vi "INI-FGV(lvlibp).vi"(4 "Raw String? (F)":bool, 5 "Write If not found?":bool, 6 "Enum":T3, 7 "Prefered Section":string, 8 "error IN":errorcluster, 9 "Path":path, 10 ">> Default Value >>":string, 11 ">> Variable Name >>":string) -> (0 "error out":errorcluster, 1 "INIConfig":T1, 2 "Key?":bool, 3 "Array":string[](array[string]))   [LabVIEW 2017, in "INI-Static-Variable-Support.lvlib"]
uses:
  INI-Static-Variable-Support.lvlib
  _fgv-oper.ctl
  LabVIEW-Config/Config.ctl
  LabVIEW-Config/LineToken.ctl
  INI-FGV.vi
  <userlib>/_NEVSTOP/Communicable State Machine(CSM)/Communicable State Machine.lvlib
  <userlib>/_NEVSTOP/Communicable State Machine(CSM)/_Shared/CSM Shared.lvlib
  LabVIEW-Config/LabVIEW-Config.lvlib
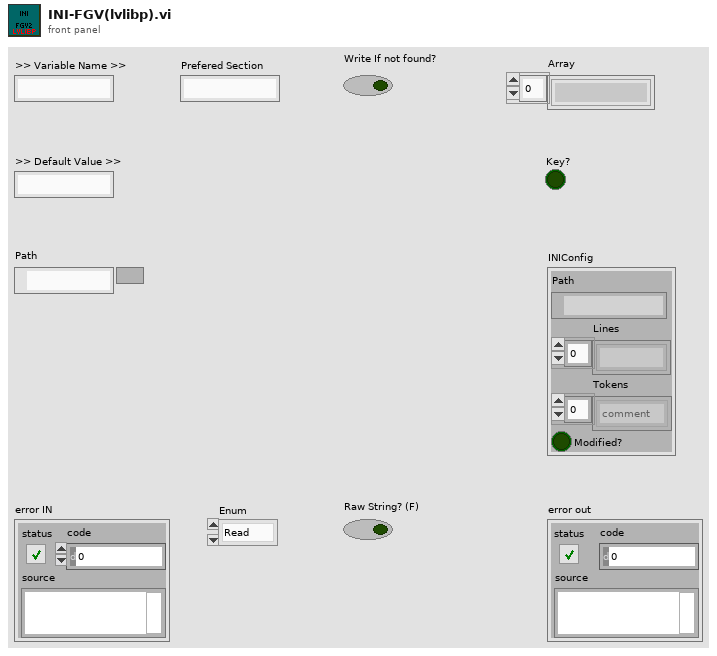
[diagram p1: front panel]
types:
  T1 = typedef "LabVIEW-Config.lvlib/Config.ctl" = cluster{"Path":path, "Lines":string[], "Tokens":T2[], "Modified?":bool}
  T2 = typedef "LabVIEW-Config.lvlib/LineToken.ctl" = enum8{"comment", "section", "key", "more"}
  T3 = typedef "INI-Static-Variable-Support.lvlib/_fgv-oper.ctl" = enum16{"Read", "Write", "Sync", "Sessions", "List Keys", "Load", "List Files", "List Variables", "List Permanent Variables", "Mark Temp Variable as Permenent", "unload", "INIConfig(Memory)", "Reset", "Restore Variable Value"}
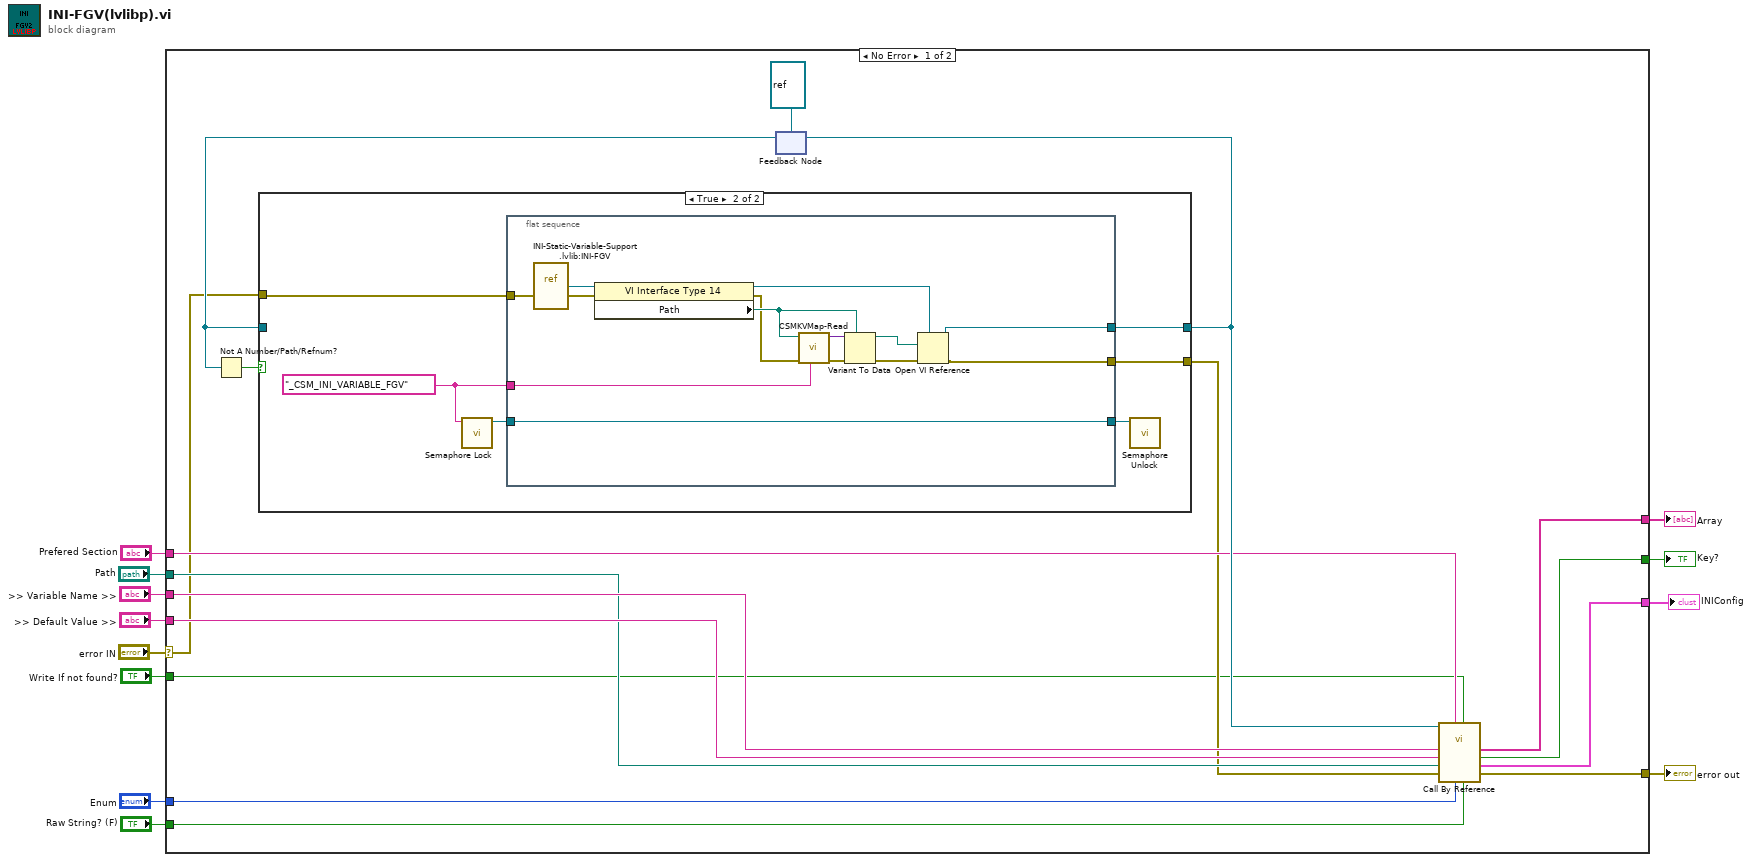
[diagram p0: block diagram]
diagram:
  n1 = case shown="No Error" "error IN" {
    selector: "error IN" -> [w20 w51]
    tunnel: ">> Default Value >>" -> [w23 _]
    tunnel: ">> Variable Name >>" -> [w24 _]
    tunnel: [w16 w51] -> w10
    tunnel: "Enum" -> [w22 _]
    tunnel: "Raw String? (F)" -> [w13 _]
    tunnel: "Write If not found?" -> [w14 _]
    tunnel: "Path" -> [w21 _]
    tunnel: "Prefered Section" -> [w25 _]
    tunnel: [w18 _] -> w3
    tunnel: [w17 _] -> w2
    tunnel: [w15 _] -> w1
    frame No Error {
      n2 = feedback #1(refnum<vi> refnum) -> (w28:refnum<vi>)
      n3 = Not A Number/Path/Refnum?(number/path/refnum=w28) -> (NaN/Path/Refnum?=w29:bool)
      n4 = case shown="True" w29 {
        tunnel: [w31 w37] -> w27
        tunnel: w28 -> [w31 _]
        tunnel: w20 -> [w30 w36]
        tunnel: [w30 w35] -> w19
        frame False {
        }
        frame True {
          w34 = "_CSM_INI_VARIABLE_FGV" ("name")
          n5 = call <userlib>:"Semaphore Lock.vi"("name"=w34) -> ("semaphore"=w33:refnum<queue>)  [unwired: 10 in]
          n6 = flat-sequence {
            tunnel: w34 -> [w46]
            tunnel: [w44] -> w37
            tunnel: w36 -> [w41]
            tunnel: [w38] -> w35
            tunnel: w33 -> [w39]
            tunnel: [w39] -> w32
            frame #0 {
              n7 = vi-ref "INI-Static-Variable-Support.lvlib:INI-FGV.vi"() -> (w43:refnum<vi>)
              n8 = property class="VI Interface Type 14"(reference=w43, error in=w41) -> (reference out=w42:refnum<vi>, error out=w40:errorcluster, "Path"=w45:path)
              n9 = call <userlib>:"CSMKVMap-Read.vi"("name"=w46, "Error in"=w40, "default value (empty variant)"=w45) -> ("Error out"=w50:errorcluster, "value"=w49:variant)  [unwired: 5 in]
              n10 = Variant To Data(error in=w50, type=w45, Variant=w49) -> (data=w48:path, error out=w47:errorcluster)
              n11 = Open VI Reference(type specifier VI Refnum (for type only)=w42, vi path=w48, error in (no error)=w47) -> (vi reference=w44:refnum<vi>, error out=w38:errorcluster)  [unwired: 3 in]
            }
          }
          n12 = call <userlib>:"Semaphore Unlock.vi"("semaphore"=w32) -> ()  [unwired: 11 in]
        }
      }
      n13 = feedback-in #1(w27) -> ()
      n14 = call-by-ref "?"(reference=w27, "Raw String? (F)"=w13, "Write If not found?"=w14, "Enum"=w22, "Prefered Section"=w25, "error IN"=w19, "Path"=w21, ">> Default Value >>"=w23, ">> Variable Name >>"=w24) -> ("error out"=w16:errorcluster, "INIConfig"=w17:T1, "Key?"=w15:bool, "Array"=w18:string[])  [unwired: 1 in, 2 out]
    }
    frame Error {
    }
  }
  "Array" <- w3
  "error out" <- w10
  "Key?" <- w1
  "INIConfig" <- w2
